vi "LUTPlane2PlaneDist.vi"(11 "ZLUT":sgl[][](array[numeric])) -> (0 "max index":i32, 1 "max diff":sgl, 2 "min index":i32, 3 "min diff":sgl, 4 "Squared diff":sgl[](array[numeric]))   [LabVIEW 2011]
panel:
  out "Squared difference":sgl[](graph)
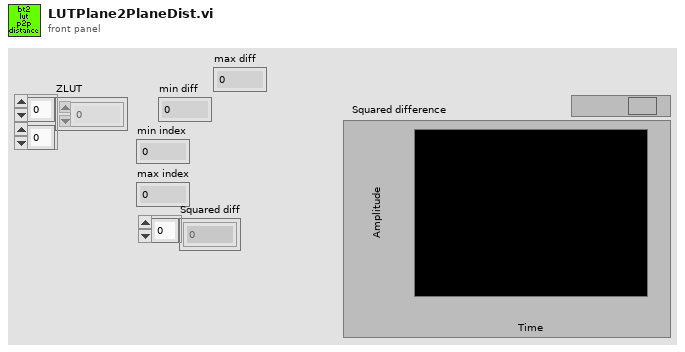
[diagram p1: front panel]
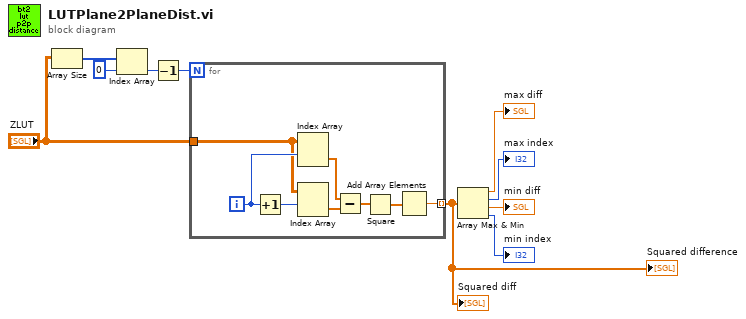
[diagram p0: block diagram]
diagram:
  n1 = Array Size(array="ZLUT") -> (size(s)=w6:i32[])
  n2 = Index Array(array=w6, index=0) -> (element=w8:i32)
  n3 = Decrement(x=w8) -> (x-1=w9:i32)
  n4 = for {
    N: w9 -> [_]
    tunnel: "ZLUT" -> [w14]
    tunnel: [w11] -> w1 mode=indexing
    i -> [w18]
    n5 = Increment(x=w18) -> (x+1=w17:i32)
    n6 = Index Array(array=w14, index (row)=w18) -> (element=w16:sgl[])  [unwired: 1 in]
    n7 = Index Array(array=w14, index (row)=w17) -> (element=w15:sgl[])  [unwired: 1 in]
    n8 = Subtract(x=w16, y=w15) -> (x-y=w13:sgl[])
    n9 = Square(x=w13) -> (x^2=w12:sgl[])
    n10 = Add Array Elements(numeric array=w12) -> (sum=w11:sgl)
  }
  "Squared diff" <- w1
  "Squared difference" <- w1
  n11 = Array Max & Min(array=w1) -> (max value=→"max diff":sgl, max index (indices)=→"max index":i32, min value=→"min diff":sgl, min index (indices)=→"min index":i32)
